vi "Calculate Rise-Fall Timing.vi"(10 "Second Pulse":waveform(dbl)={"t0"=timestamp(0 s since 1904-01-01), "dt"=0.0, "Y"=[]}, 11 "First Pulse":waveform(dbl)={"t0"=timestamp(0 s since 1904-01-01), "dt"=0.0, "Y"=[]}) -> (3 "Time Difference":dbl)   [LabVIEW 2010]
uses:
  <vilib>/measure/mascope.llb/Amplitude and Levels 1 chan.vi
  <vilib>/measure/mamon.llb/Trigger Detection for 1 Channel.vi
  <vilib>/measure/NI_MAPro.lvlib
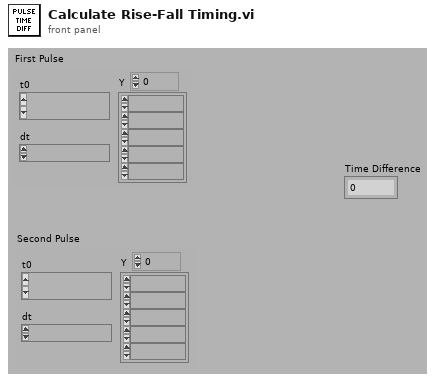
[diagram p1: front panel]
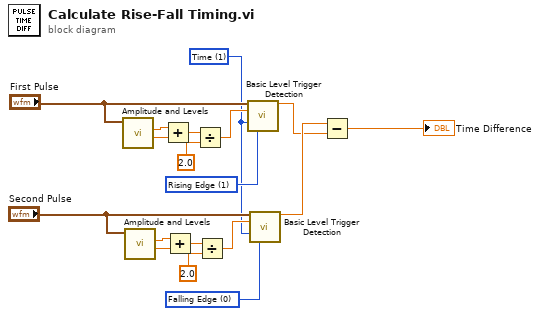
[diagram p0: block diagram]
diagram:
  w4 = u16 1 items=["Index", "Time"] ("location mode")
  w5 = u16 0 items=["Falling Edge", "Rising Edge"] ("trigger slope")
  w6 = u16 1 items=["Falling Edge", "Rising Edge"] ("trigger slope")
  n1 = call-poly <vilib>:"Amplitude and Levels.vi"("signal in"="First Pulse") -> ("low state level"=w16:dbl, "high state level"=w17:dbl)  [unwired: 7 in, 2 out]
  n2 = call-poly <vilib>:"Amplitude and Levels.vi"("signal in"="Second Pulse") -> ("low state level"=w11:dbl, "high state level"=w12:dbl)  [unwired: 7 in, 2 out]
  n3 = Add(x=w17, y=w16) -> (x+y=w15:dbl)
  n4 = Add(x=w12, y=w11) -> (x+y=w10:dbl)
  n5 = Divide(x=w15, y=2.0) -> (x/y=w13:dbl)
  n6 = Divide(x=w10, y=2.0) -> (x/y=w8:dbl)
  n7 = call-poly <vilib>:"Basic Level Trigger Detection.vi"("signal in"="First Pulse", "level"=w13, "location mode"=w4, "trigger slope"=w6) -> ("trigger location"=w2:dbl)  [unwired: 9 in, 2 out]
  n8 = call-poly <vilib>:"Basic Level Trigger Detection.vi"("signal in"="Second Pulse", "level"=w8, "location mode"=w4, "trigger slope"=w5) -> ("trigger location"=w3:dbl)  [unwired: 9 in, 2 out]
  n9 = Subtract(x=w3, y=w2) -> (x-y=→"Time Difference":dbl)
